vi "ex5-10.vi"() -> ()   [LabVIEW 2014]
uses:
  <vilib>/NXT/Subs/MotorOutput.ctl
  <vilib>/NXT/Dual Mode Library/Motors/ResetMotor.vi
  <vilib>/NXT/Dual Mode Library/Motors/Rotation.vi
  <vilib>/NXT/Dual Mode Library/Motors/MotorOn.vi
panel:
  out "期望角度":dbl
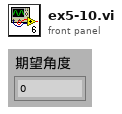
[diagram p1: front panel]
types:
  T1 = typedef "MotorOutput.ctl" = u8
  T2 = typedef "LVHSConnector.ctl" = refnum<class "BrickReference.lvclass">
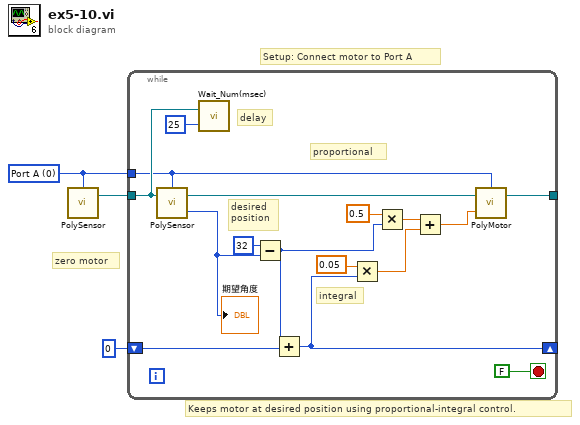
[diagram p0: block diagram]
diagram:
  w3 = T1 0 items=["Port A", "Port B", "Port C", "All Ports"] ("Output Port")
  # "zero motor"
  # "Keeps motor at desired position using proportional-integral control."
  # "Setup: Connect motor to Port A"
  n1 = call-poly <vilib>:"PolySensor.vi"("Port (All Ports)"=w3) -> ("NXT/EV3"=w2:T2)  [unwired: 1 in, 2 out]
  n2 = while {
    shift-right: [w14] -> _
    shift-left: 0 ("RotationCount") -> [w18]
    tunnel: w3 -> [w6]
    tunnel: w2 -> [w7]
    tunnel: [w9] -> _
    stop <- FALSE stop-if-true
    # "integral"
    # "proportional"
    # "desired\nposition"
    # "delay"
    n3 = call-poly <vilib>:"PolySensor.vi"("NXT/EV3"=w7, "Port (Port A)"=w6) -> ("Angle of Rotation"=w4:i32, "NXT/EV3"=w10:T2)  [unwired: 1 out]
    "期望角度" <- w4
    n4 = call <vilib>:"Wait_Num(msec).vi"("Time (100 msec)"=u32 25 ("milliseconds to wait"), "NXT/EV3"=w7) -> ()  [unwired: 2 in, 1 out]
    n5 = Subtract(x=32, y=w4) -> (x-y=w15:i32)
    n6 = Add(x=w15, y=w18) -> (x+y=w14:i32)
    n7 = Multiply(x=0.05, y=w14) -> (x*y=w12:dbl)
    n8 = Multiply(x=0.5 ("y"), y=w15) -> (x*y=w17:dbl)
    n9 = Add(x=w17, y=w12) -> (x+y=w11:dbl)
    n10 = call-poly <vilib>:"PolyMotor.vi"("Power (75)"=w11, "NXT/EV3"=w10, "Output Port (All Ports)"=w6) -> ("NXT/EV3"=w9:T2)  [unwired: 1 out]
  }
